vi "SandBox - Show Main VI.vi"   [LabVIEW 2016]
uses:
  <vilib>/regexp/Match Regular Expression.xnode
types:
  T1 = enum32{"Invalid", "Standard", "Closed", "Hidden", "Minimized", "Maximized"}
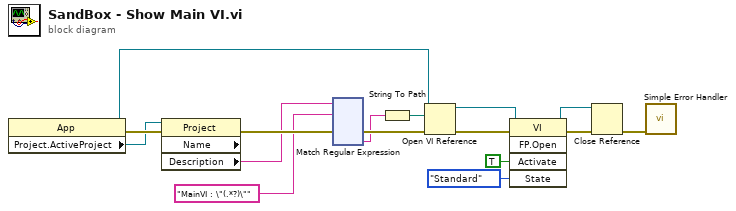
[diagram p0: block diagram]
diagram:
  n1 = property class="App"() -> (reference out=w7:refnum<vi>, error out=w16:errorcluster, "Project.ActiveProject"=w15:refnum<vi>)  [unwired: 2 in]
  n2 = property class="Project" props=["Name", "Description"](reference=w15, error in=w16) -> (error out=w14:errorcluster, "Description"=w13:string)  [unwired: 2 out]
  n3 = xnode "Match Regular Expression"("input string"=w13, "regular expression"="MainVI : \"(.*?)\"", "error in"=w14) -> ("error out"=w11:errorcluster, "submatch 1"=w6:string)  [unwired: 3 in, 4 out]
  n4 = String To Path(string=w6) -> (path=w1:path)
  n5 = Open VI Reference(application reference (local)=w7, vi path=w1, error in (no error)=w11) -> (vi reference=w5:refnum<vi>, error out=w10:errorcluster)  [unwired: 3 in]
  n6 = invoke class="VI" method="FP.Open"(reference=w5, error in=w10, "Activate"=TRUE ("Activate?"), "State"=T1."Standard") -> (reference out=w4:refnum<vi>, error out=w9:errorcluster)  [unwired: 1 in, 3 out]
  n7 = Close Reference(reference=w4, error in (no error)=w9) -> (error out=w8:errorcluster)
  n8 = call <vilib>:"Simple Error Handler.vi"("error in (no error)"=w8) -> ()  [unwired: 4 in, 5 out]
